vi "Xylo_Essai_3_Efficace.vi"() -> ()   [LabVIEW 2018]
panel:
  in  "Open Button":bool
  in  "Save As Button":bool
  out "tableauRythme":u8[](array[numeric])
  in  "Rythme Choix":string(combo)
  in  "RESET Button":bool
  out "tableauNotes":u8[](array[numeric])
  in  "stop":bool
  out "Numeric":i32
  in  "Array":bool[](array[boolean])=[FALSE, FALSE, FALSE, FALSE, FALSE, FALSE, FALSE, FALSE] caption="Clavier"
  out "Messure Musicale":dbl(graph)
  in  "File Path Control 2":path
  in  "Save Button":bool
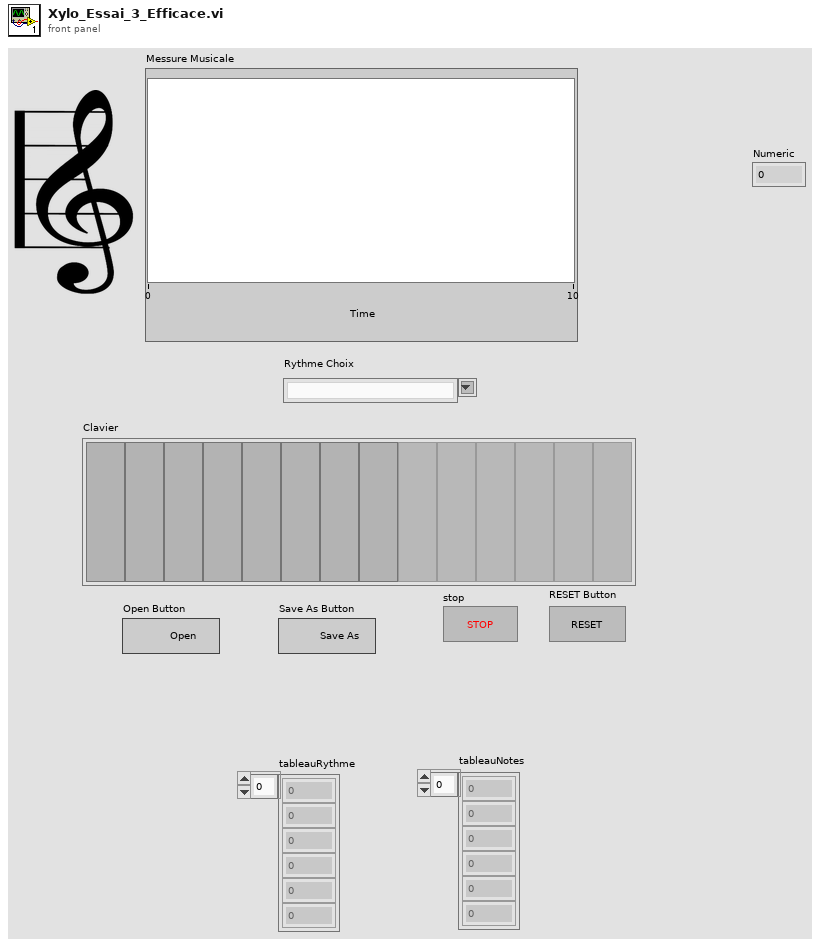
[diagram p1: front panel]
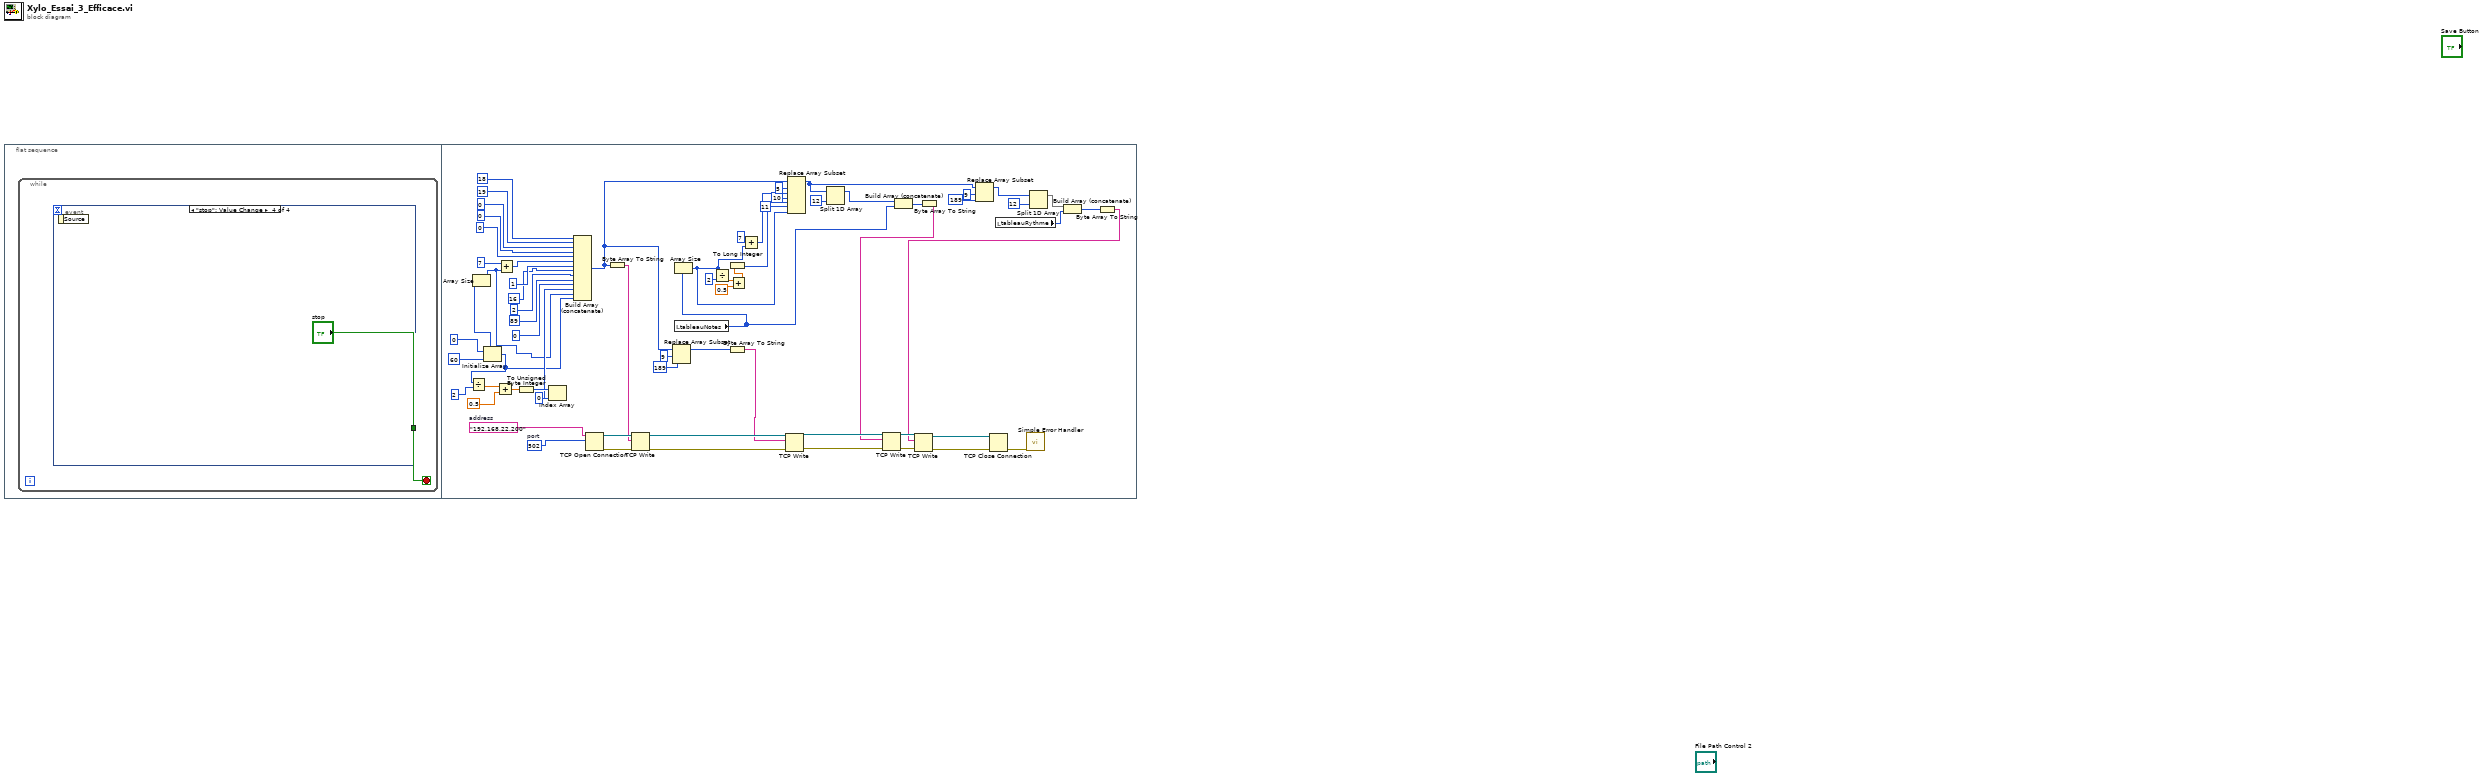
[diagram p0: block diagram]
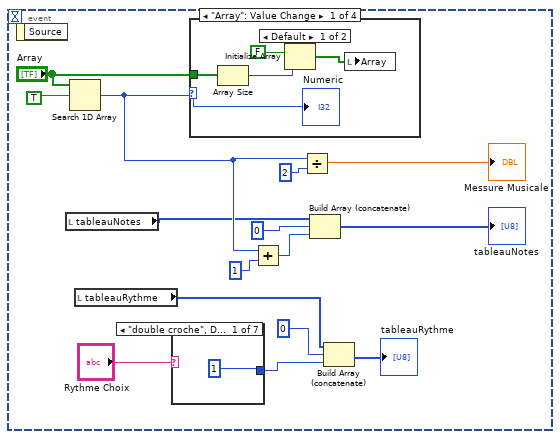
[diagram p2: hidden frame]
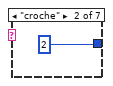
[diagram p3: hidden frame]
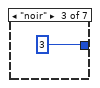
[diagram p4: hidden frame]
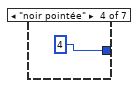
[diagram p5: hidden frame]
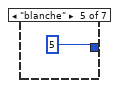
[diagram p6: hidden frame]
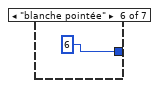
[diagram p7: hidden frame]
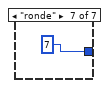
[diagram p8: hidden frame]
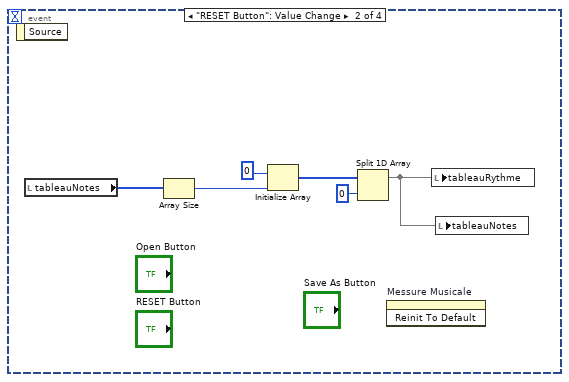
[diagram p10: hidden frame]
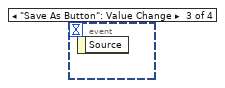
[diagram p11: hidden frame]
diagram:
  n1 = flat-sequence {
    frame #0 {
      n2 = while {
        stop <- w1 stop-if-true
        n3 = event shown="[3] \"stop\": Value Change" {
          selector: _ -> [_ _ _ _]
          dyn-events: _ -> [_ _ _ _]
          timeout: _ -> [_ _ _ _]
          tunnel: [_ _ _ "stop"] -> w1
          event "Array": Value Change {
            n4 = event-data() -> ()  [unwired: 1 in, 1 out]
            n5 = local read "tableauNotes"() -> (w10:u8[])
            n6 = Search 1D Array(1D array="Array", element=TRUE) -> (index of element=w12:i32)  [unwired: 1 in]
            n7 = local read "tableauRythme"() -> (w2:u8[])
            n8 = case shown="\"double croche\", Default" "Rythme Choix" {
              tunnel: [1 2 3 4 5 6 7] -> w4
              frame "double croche", Default {
              }
              frame "croche" {
              }
              frame "noir" {
              }
              frame "noir pointée" {
              }
              frame "blanche" {
              }
              frame "blanche pointée" {
              }
              frame "ronde" {
              }
            }
            n9 = case shown="Default" w12 {
              selector: w12 -> [w25 _]
              tunnel: "Array" -> [w26 _]
              frame Default {
                n10 = Array Size(array=w26) -> (size(s)=w28:i32)
                n11 = Initialize Array(FALSE ("element"), w28) -> (w24:bool[])
                n12 = local write "Array"(w24) -> ()
                "Numeric" <- w25
              }
              frame -1 {
              }
            }
            n13 = Add(x=w12, y=1) -> (x+y=w9:i32)
            n14 = Divide(x=w12, y=2 ("Numeric")) -> (x/y=→"Messure Musicale":dbl)
            n15 = Build Array (concatenate)(w10, 0 ("element"), w9) -> (→"tableauNotes":i32[])
            n16 = Build Array (concatenate)(w2, 0 ("element"), w4) -> (→"tableauRythme":i32[])
          }
          event "RESET Button": Value Change {
            n17 = event-data() -> ()  [unwired: 1 in, 1 out]
            n18 = local read "tableauNotes"() -> (w33:u8[])
            n19 = Array Size(array=w33) -> (size(s)=w32:i32)
            n20 = Initialize Array(u8 0 ("element"), w32) -> (w31:u8[])
            n21 = Split 1D Array(array=w31, index=0) -> (first subarray=w29:u8[])  [unwired: 1 out]
            n22 = invoke on="Messure Musicale" class="WFChart (strict)" method="Reinit To Default"() -> ()  [unwired: 3 in, 3 out]
            n23 = local write "tableauRythme"(w29) -> ()
            n24 = local write "tableauNotes"(w29) -> ()
          }
          event "Save As Button": Value Change {
            n25 = event-data() -> ()  [unwired: 1 in, 1 out]
          }
          event "stop": Value Change {
            n26 = event-data() -> ()  [unwired: 1 in, 1 out]
          }
        }
      }
    }
    frame #1 {
      w100 = "192.168.22.200"  # address
      w101 = 502  # port
      n27 = Initialize Array(u8 0 ("element"), 60 ("dimension size")) -> (w36:u8[])
      n28 = Divide(x=w36, y=2) -> (x/y=w77:dbl[])
      n29 = Array Size(array=w36) -> (size(s)=w37:i32)
      n30 = Add(x=w77, y=0.5) -> (x+y=w78:dbl[])
      n31 = Add(x=7, y=w37) -> (x+y=w81:i32)
      n32 = To Unsigned Byte Integer(number=w78) -> (unsigned 8bit integer=w62:u8[])
      n33 = Index Array(array=w62, index=0) -> (element=w38:u8)
      n34 = Build Array (concatenate)(18, 19, 0, 0, 0, w81, 1, 16, 2, 89, 0, w38, w37, w36) -> (w70:i32[])
      n35 = TCP Open Connection(address=w100, remote port or service name=w101) -> (connection ID=w95:refnum<k5>, error out=w92:errorcluster)  [unwired: 3 in]
      n36 = Byte Array To String(unsigned byte array=w70) -> (string=w75:string)
      n37 = TCP Write(connection ID=w95, data in=w75, error in (no error)=w92) -> (connection ID out=w94:refnum<k5>, error out=w91:errorcluster)  [unwired: 1 in, 1 out]
      n38 = Replace Array Subset(array=w70, new element=189 ("new element/subarray"), index=9) -> (w72:i32[])
      n39 = local read "tableauNotes"() -> (w64:u8[])
      n40 = Array Size(array=w64) -> (size(s)=w54:i32)
      n41 = Divide(x=w54, y=2) -> (x/y=w67:dbl)
      n42 = Byte Array To String(unsigned byte array=w72) -> (string=w71:string)
      n43 = Add(x=w67, y=0.5) -> (x+y=w60:dbl)
      n44 = To Long Integer(number=w60) -> (32bit integer=w56:i32)
      n45 = Add(x=7, y=w54) -> (x+y=w59:i32)
      n46 = TCP Write(connection ID=w94, data in=w71, error in (no error)=w91) -> (connection ID out=w93:refnum<k5>, error out=w90:errorcluster)  [unwired: 1 in, 1 out]
      n47 = Replace Array Subset(array=w70, new element #1=w59, index #1=5 ("index"), new element #2=w56, index #2=10 ("index"), new element #3=w54, index #3=11 ("index")) -> (w46:i32[])
      n48 = Split 1D Array(array=w46, index=12) -> (first subarray=w63:i32[])  [unwired: 1 out]
      n49 = Build Array (concatenate)(w63, w64) -> (w53:i32[])
      n50 = Byte Array To String(unsigned byte array=w53) -> (string=w52:string)
      n51 = TCP Write(connection ID=w93, data in=w52, error in (no error)=w90) -> (connection ID out=w99:refnum<k5>, error out=w98:errorcluster)  [unwired: 1 in, 1 out]
      n52 = Replace Array Subset(array=w46, new element=189 ("new element/subarray"), index=9) -> (w43:i32[])
      n53 = local read "tableauRythme"() -> (w49:u8[])
      n54 = Split 1D Array(array=w43, index=12) -> (first subarray=w50:i32[])  [unwired: 1 out]
      n55 = Build Array (concatenate)(w50, w49) -> (w48:i32[])
      n56 = Byte Array To String(unsigned byte array=w48) -> (string=w47:string)
      n57 = TCP Write(connection ID=w99, data in=w47, error in (no error)=w98) -> (connection ID out=w96:refnum<k5>, error out=w97:errorcluster)  [unwired: 1 in, 1 out]
      n58 = TCP Close Connection(connection ID=w96, error in (no error)=w97) -> (error out=w102:errorcluster)  [unwired: 1 in, 1 out]
      n59 = call <vilib>:"Simple Error Handler.vi"("error in (no error)"=w102) -> ()  [unwired: 4 in, 5 out]
    }
  }
